vi "Create Evaluations.vi"(8 "error in (no error)":errorcluster, 11 "IEvaluation in":refnum<class "ET_Delay_Sweep.lvclass">) -> (0 "error out":errorcluster, 2 "Evaluations Out":T1[](array[typedef]) {"Low Limit" format="%#_13g"; "SI Scaling" items=["femto"=-15, "pico"=-12, "nano"=-9, "micro"=-6, "milli"=-3, "percent"=-2, ""=0, "kilo"=3, "mega"=6, "giga"=9, "tera"=12]}, 3 "IEvaluation out":refnum<class "ET_Delay_Sweep.lvclass">)   [LabVIEW 2016, in "SeqAuto Evaluations.lvlib" / "ET_Delay_Sweep.lvclass"]
uses:
  ET_Delay_Sweep.lvclass
  C:/projects/STS/Common/Sequence Automation/Plugins/SeqAuto IEvaluation.lvlibp/SeqAuto IEvaluation.lvclass
  Plugins/TestStand API Tools (TSAT).lvlibp/Evaluation Actions/Includes/Controls/TSAT Evaluation.ctl
  Plugins/TestStand API Tools (TSAT).lvlibp/Evaluation Actions/Includes/Controls/TSAT Eval SI Unit Scaling.ctl
  Plugins/TestStand API Tools (TSAT).lvlibp/Evaluation Actions/Includes/Controls/TSAT Evaluation Type.ctl
  ET_Delay_Sweep.lvclass/ET_Delay_Sweep.ctl
  Plugins/SeqAuto IEvaluation.lvlibp/Read Measurement Name.vi
  Plugins/TestStand API Tools (TSAT).lvlibp/Evaluation Actions/TSAT Evaluation Actions.lvlib
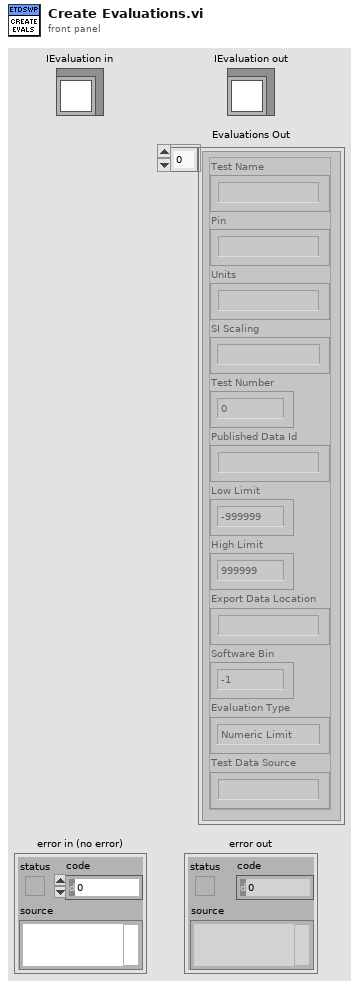
[diagram p1: front panel]
types:
  T1 = typedef "TestStand API Tools (TSAT).lvlibp/TSAT Evaluation Actions.lvlib/TSAT Evaluation.ctl" = cluster{"Test Name":string, "Pin":string, "Units":string, "SI Scaling":T2, "Test Number":i32, "Published Data Id":string, "Low Limit":dbl, "High Limit":dbl, "Export Data Location":string, "Software Bin":i64, "Evaluation Type":T3, "Test Data Source":string}
  T2 = typedef "TestStand API Tools (TSAT).lvlibp/TSAT Evaluation Actions.lvlib/TSAT Eval SI Unit Scaling.ctl" = i16
  T3 = typedef "TestStand API Tools (TSAT).lvlibp/TSAT Evaluation Actions.lvlib/TSAT Evaluation Type.ctl" = enum16{"Numeric Limit", "Pass/Fail", "None"}
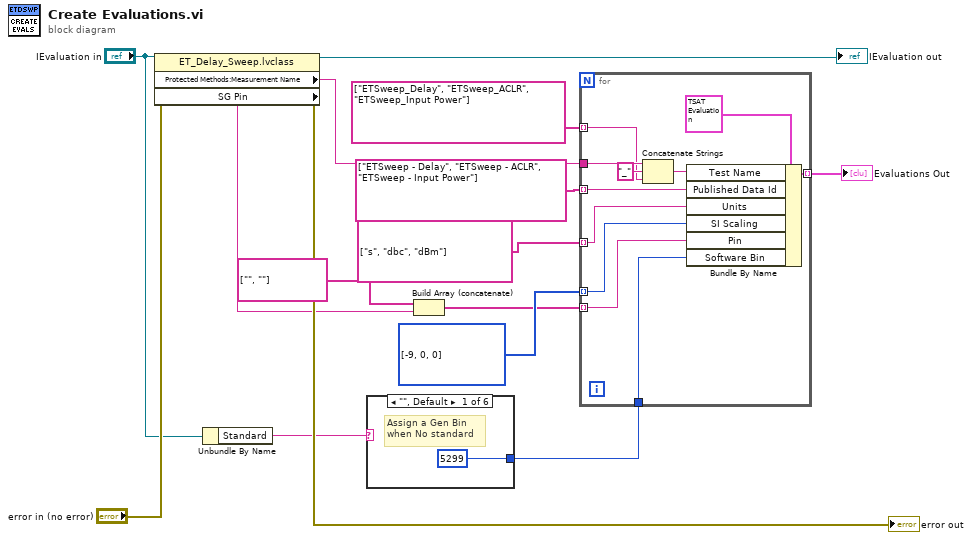
[diagram p0: block diagram]
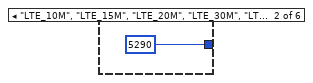
[diagram p2: hidden frame]
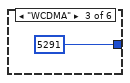
[diagram p3: hidden frame]
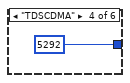
[diagram p4: hidden frame]
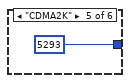
[diagram p5: hidden frame]
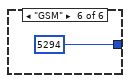
[diagram p6: hidden frame]
diagram:
  w8 = T2[] [-9, 0, 0] items=["femto"=-15, "pico"=-12, "nano"=-9, "micro"=-6, "milli"=-3, "percent"=-2, ""=0, "kilo"=3, "mega"=6, "giga"=9, "tera"=12]
  n1 = property class="ET_Delay_Sweep.lvclass"(reference="IEvaluation in", error in="error in (no error)") -> (reference out=→"IEvaluation out":refnum<class "ET_Delay_Sweep.lvclass">, error out=→"error out":errorcluster, "Protected Methods:Measurement Name"=w11:string, "SG Pin"=w5:string)
  n2 = Unbundle By Name("IEvaluation in") -> ("Standard"=w2:string)
  n3 = case shown="\"\", Default" w2 {
    tunnel: [i64 5299 ("Software Bin") i64 5290 ("Software Bin") i64 5291 ("Software Bin") i64 5292 ("Software Bin") i64 5293 ("Software Bin") i64 5294 ("Software Bin")] -> w1
    frame "", Default {
      # "Assign a Gen Bin\nwhen No standard"
    }
    frame "LTE_10M", "LTE_15M", "LTE_20M", "LTE_30M", "LTE_40M" {
    }
    frame "WCDMA" {
    }
    frame "TDSCDMA" {
    }
    frame "CDMA2K" {
    }
    frame "GSM" {
    }
  }
  n4 = Build Array (concatenate)(string[] ["", ""], w5) -> (w4:string[])
  n5 = for {
    tunnel: [w31] -> w14 mode=indexing
    tunnel: w11 -> [w30]
    tunnel: string[] ["ETSweep_Delay", "ETSweep_ACLR", "ETSweep_Input Power"] -> [w26] mode=indexing
    tunnel: string[] ["s", "dbc", "dBm"] -> [w27] mode=indexing
    tunnel: w8 -> [w25] mode=indexing
    tunnel: string[] ["ETSweep - Delay", "ETSweep - ACLR", "ETSweep - Input Power"] -> [w24] mode=indexing
    tunnel: w4 -> [w23] mode=indexing
    tunnel: w1 -> [w22]
    n6 = Concatenate Strings(w30, "_" ("string"), w26) -> (w29:string)
    n7 = Bundle By Name(cluster=T1 {"Test Name"="", "Pin"="", "Units"="", "SI Scaling"=0, "Test Number"=0, "Published Data Id"="", "Low Limit"=-999999.0, "High Limit"=999999.0, "Export Data Location"="", "Software Bin"=-1, "Evaluation Type"=enum."Numeric Limit", "Test Data Source"=""} ("Evaluation"), "Test Name"=w29, "Published Data Id"=w24, "Units"=w27, "SI Scaling"=w25, "Pin"=w23, "Software Bin"=w22) -> (w31:T1)
  }
  "Evaluations Out" <- w14
